vi "Enable Math Operation.vi"(8 "error in (no error)":errorcluster, 9 "Enable Math Operations (F:Disable)":bool, 10 "Function (0: Volts)":u16(ring) items=["Volts", "Current", "Resistance", "Digitize Voltage", "Digitize Current"], 11 "VISA resource name":refnum<visa-resource-name>) -> (0 "error out":errorcluster, 3 "VISA resource name out":refnum<visa-resource-name>)   [LabVIEW 2020, in "Keithley 2450.lvlib"]
doc: "Enables or Disables math operation."
uses:
  Keithley 2450.lvlib
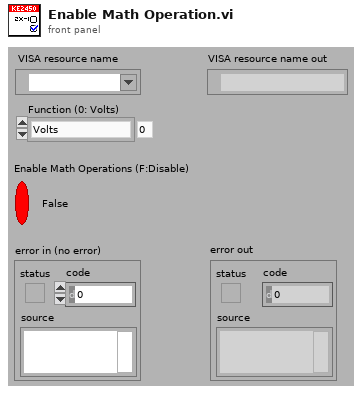
[diagram p1: front panel]
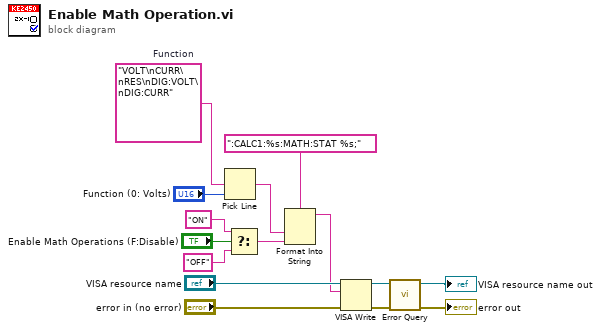
[diagram p0: block diagram]
diagram:
  w9 = "VOLT\nCURR\nRES\nDIG:VOLT\nDIG:CURR"  # Function
  n1 = Pick Line(multi-line string=w9, line index="Function (0: Volts)") -> (output string=w3:string)  [unwired: 1 out]
  n2 = Select(t="ON" ("format string"), s="Enable Math Operations (F:Disable)", f="OFF" ("format string")) -> (s? t:f=w2:string)
  n3 = Format Into String(format string=":CALC1:%s:MATH:STAT %s;", w3, w2) -> (resulting string=w1:string)  [unwired: 2 in, 1 out]
  n4 = VISA Write(VISA resource name="VISA resource name", write buffer=w1, error in (no error)="error in (no error)") -> (VISA resource name out=w13:refnum<visa-resource-name>, error out=w10:errorcluster)  [unwired: 1 out]
  n5 = call "Error Query.vi"("error in (no error)"=w10, "VISA resource name"=w13) -> ("error out"=→"error out":errorcluster, "VISA resource name out"=→"VISA resource name out":refnum<visa-resource-name>)  [unwired: 8 out]
